vi "UpdateEncoder.vi"(8 "Steps":i8, 9 "Address":i32, 10 "Code67Memory":refnum<k21>, 11 "Code66Memory":refnum<k21>) -> ()   [LabVIEW 2016, in "FPGAMockMDILC.lvlib"]
uses:
  FPGAMockMDILC.lvlib
  <vilib>/rvi/Emulation/niFpgaSctlEmulationGetInTimedLoop.vi
  <vilib>/Utility/error.llb/Clear Errors.vi
  <vilib>/rvi/DataTransferAndStorage/Container/Common/niFpgaContainerExecOnDevCompGetState.vi
  <vilib>/rvi/Emulation/niFpgaEmulationIsFPGAContextNoSignature.vi
  <vilib>/rvi/DataTransferAndStorage/Container/Common/niFpgaContainerGetUniqueNameForEmu.vi
  <vilib>/rvi/Emulation/niFpgaProcessEmulError.vi
  <vilib>/rvi/errors/nirviReportUnexpectedCaseInternalError (U32).vi
  <vilib>/rvi/Memory/Memory_Emulation/niFpgaMemoryEmulationCacheClearOnFirstRun.vi
  <vilib>/rvi/Memory/Memory_Emulation/nirvimemoryEmulationManagerCache_MakeExclusive.vi
  <vilib>/rvi/Memory/Memory_Emulation/niFpgaMemoryEmulationValidateCache.vi
  <vilib>/rvi/Memory/Memory_Emulation/nirvimemoryEmulationManagerCache_InsertValue.vi
  <vilib>/rvi/Memory/Memory_Emulation/nirvimemoryEmulationManagerCache_ReleaseExclusive.vi
  <vilib>/rvi/Memory/Memory_Emulation/nirvimemoryEmulationManagerCache_GetValue.vi
  <vilib>/rvi/Memory/Memory_Emulation/nirvimemoryEmulationManagerCache_SetValue.vi
  <vilib>/rvi/Emulation/niFpgaSctlEmulationResourceMgr.vi
  <vilib>/rvi/DataTransferAndStorage/Container/XNode/niFpgaContainer.xnode
  <vilib>/rvi/Memory/Memory_Emulation/niFpgaMemoryEmulationRefIn.vi
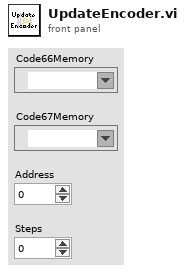
[diagram p1: front panel]
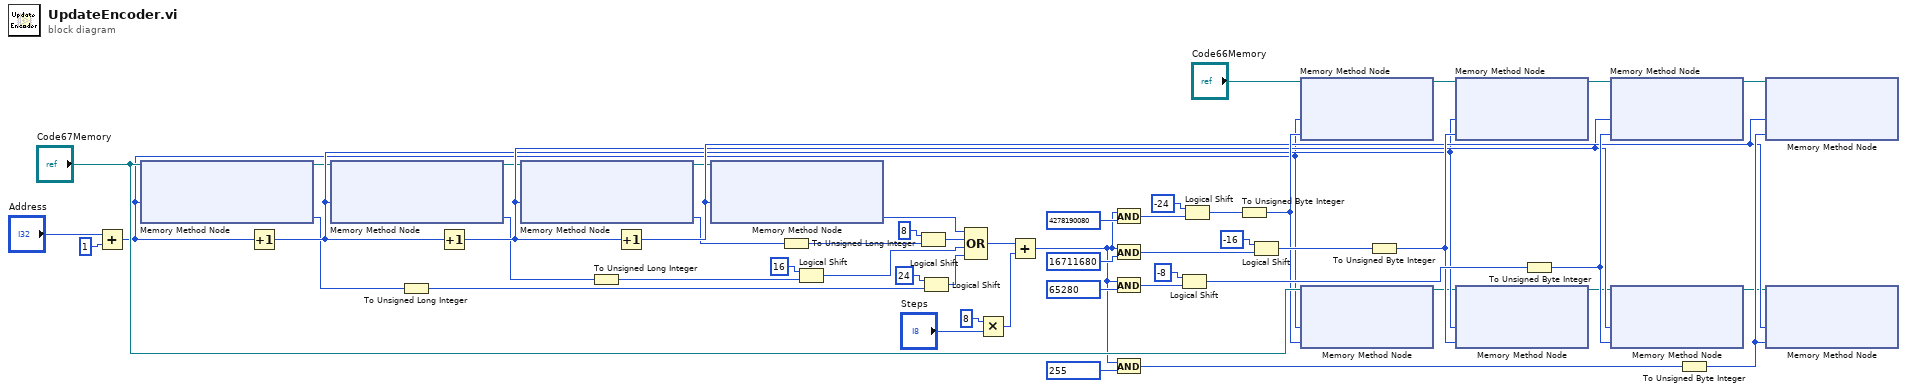
[diagram p0: block diagram]
diagram:
  n1 = Add(x="Address", y=1) -> (x+y=w35:i32)
  n2 = xnode ("Memory Method Node")("Address"=w35, "Memory In"="Code67Memory") -> ("Data"=w4:u8, "Memory Out"=w1:refnum<k21>)
  n3 = Increment(x=w35) -> (x+1=w37:i32)
  n4 = xnode ("Memory Method Node")("Address"=w37, "Memory In"=w1) -> ("Data"=w9:u8, "Memory Out"=w13:refnum<k21>)
  n5 = To Unsigned Long Integer(number=w4) -> (unsigned 32bit integer=w5:u32)
  n6 = Increment(x=w37) -> (x+1=w39:i32)
  n7 = xnode ("Memory Method Node")("Address"=w39, "Memory In"=w13) -> ("Data"=w12:u8, "Memory Out"=w14:refnum<k21>)
  n8 = To Unsigned Long Integer(number=w9) -> (unsigned 32bit integer=w8:u32)
  n9 = Increment(x=w39) -> (x+1=w41:i32)
  n10 = xnode ("Memory Method Node")("Address"=w41, "Memory In"=w14) -> ("Data"=w18:u8)  [unwired: 1 out]
  n11 = To Unsigned Long Integer(number=w12) -> (unsigned 32bit integer=w10:u32)
  n12 = Logical Shift(y=i16 16, x=w8) -> (x << y=w16:u32)
  n13 = Logical Shift(y=i16 8, x=w10) -> (x << y=w17:u32)
  n14 = Logical Shift(y=i16 24, x=w5) -> (x << y=w15:u32)
  n15 = Compound Arithmetic op=OR(w18, w17, w16, w15) -> (w19:u32)
  n16 = Multiply(x=8 ("y"), y="Steps") -> (x*y=w52:i32)
  n17 = Add(x=w19, y=w52) -> (x+y=w20:u32)
  n18 = And(x=w20, y=u32 4278190080) -> (x .and. y?=w25:u32)
  n19 = And(x=w20, y=u32 16711680) -> (x .and. y?=w26:u32)
  n20 = And(x=w20, y=u32 65280) -> (x .and. y?=w27:u32)
  n21 = And(x=w20, y=u32 255) -> (x .and. y?=w42:u32)
  n22 = Logical Shift(y=i16 -8, x=w27) -> (x << y=w48:u32)
  n23 = Logical Shift(y=i16 -24, x=w25) -> (x << y=w44:u32)
  n24 = To Unsigned Byte Integer(number=w44) -> (unsigned 8bit integer=w45:u8)
  n25 = Logical Shift(y=i16 -16, x=w26) -> (x << y=w46:u32)
  n26 = xnode ("Memory Method Node")("Address"=w35, "Data"=w45, "Memory In"="Code66Memory") -> ("Memory Out"=w32:refnum<k21>)
  n27 = xnode ("Memory Method Node")("Address"=w35, "Data"=w45, "Memory In"="Code67Memory") -> ("Memory Out"=w36:refnum<k21>)
  n28 = To Unsigned Byte Integer(number=w46) -> (unsigned 8bit integer=w47:u8)
  n29 = xnode ("Memory Method Node")("Address"=w37, "Data"=w47, "Memory In"=w32) -> ("Memory Out"=w33:refnum<k21>)
  n30 = xnode ("Memory Method Node")("Address"=w37, "Data"=w47, "Memory In"=w36) -> ("Memory Out"=w38:refnum<k21>)
  n31 = To Unsigned Byte Integer(number=w48) -> (unsigned 8bit integer=w49:u8)
  n32 = xnode ("Memory Method Node")("Address"=w39, "Data"=w49, "Memory In"=w33) -> ("Memory Out"=w34:refnum<k21>)
  n33 = xnode ("Memory Method Node")("Address"=w39, "Data"=w49, "Memory In"=w38) -> ("Memory Out"=w40:refnum<k21>)
  n34 = To Unsigned Byte Integer(number=w42) -> (unsigned 8bit integer=w43:u8)
  n35 = xnode ("Memory Method Node")("Address"=w41, "Data"=w43, "Memory In"=w34) -> ()  [unwired: 1 out]
  n36 = xnode ("Memory Method Node")("Address"=w41, "Data"=w43, "Memory In"=w40) -> ()  [unwired: 1 out]
